vi "simulado.vi"() -> ()   [LabVIEW 2011]
uses:
  <vilib>/Simulation/Scripting/Companion Diagram/SimConfigNode/SimParams.ctl
  <vilib>/Simulation/Scripting/Companion Diagram/SimConfigNode/_simSolvers.ctl
  <vilib>/Simulation/Implementation/Shared/SIMSCR Execution Mode.ctl
  <vilib>/Simulation/Param Hierarchy/Typedefs/SIMPH Param Control Actions.ctl
  <vilib>/Simulation/Implementation/Shared/NILVSim_FinalizeModel.vi
  <vilib>/Simulation/DiscreteLinear/Implementation/NILVSim Discrete Transfer Function Direct.llb/SIM Discrete Transfer Function Direct (SISO CD).vi
  <vilib>/Simulation/DiscreteLinear/Implementation/NILVSim Discrete ZOH.llb/SIM Discrete ZOH (scalar).vi
  <vilib>/Simulation/Nonlinear/Implementation/NILVSim Saturation.llb/SIM Saturation (scalar).vi
  <vilib>/Simulation/SignalDisplay/Implementation/NILVSim Time Waveform.llb/SIM Time Waveform (vector).vi
  <vilib>/Simulation/Utility/Implementation/SIM Halt.vi
  <vilib>/Simulation/ContinuousLinear/Implementation/NILVSim Transfer Function.llb/SIM Transfer Function Collector (SISO).vi
  <vilib>/Simulation/ContinuousLinear/Implementation/NILVSim Transfer Function.llb/SIM Transfer Function Distributor (SISO CD).vi
  <vilib>/Simulation/Implementation/Shared/NILVSim_Manager.vi
  <vilib>/Simulation/Implementation/Shared/NILVSim_ParamChanged.vi
  <vilib>/Simulation/Utility/Implementation/NILVSim Get Time and IsAcceptedStep.vi
  <vilib>/addons/Control Design/_Model Construction/Model Creation.llb/Model Creation SubVI/cd_Create Transfer Function Model.vi
  <vilib>/addons/Control Design/_Utility/Model Viewer.llb/Model Viewer SubVI/cd_Draw Transfer Function Equation (TF).vi
  <vilib>/Simulation/Implementation/Shared/SIM Unbundle Sim Info.vi
  <vilib>/Simulation/Implementation/Shared/NILVSim_GetModelError.vi
  <vilib>/Simulation/Implementation/Shared/SIM Bundle Sim Info.vi
  <vilib>/Simulation/Implementation/Shared/NILVSim_Initialize.vi
  <vilib>/Simulation/Scripting/Companion Diagram/SimConfigNode/SimDog.xnode
  <vilib>/Simulation/Implementation/XNodeFramework/SimXNode/SimX.xnode
  <vilib>/addons/Control Design/_Model Construction/Model Typedefs.llb/CD Transfer Function Model (MIMO).ctl
  <vilib>/addons/Control Design/_Model Construction/Model Typedefs.llb/CD General Elements.ctl
  <vilib>/addons/Control Design/_Model Construction/Model Typedefs.llb/CD Transfer Function Model (SISO).ctl
  <vilib>/addons/Control Design/_Model Construction/NI_LinSys_Model Creation.lvlib
  <vilib>/addons/Control Design/_Utility/NI_CD_Model Viewer.lvlib
  <vilib>/addons/Control Design/_Model Construction/NI_LinSys_Model Typedefs.lvlib
  <vilib>/Simulation/ContinuousLinear/Implementation/NILVSim Transfer Function.llb/SIM Transfer Function (SISO CD).vi
  <vilib>/Simulation/Implementation/Shared/NI_SIM_Implementation.lvlib
panel:
  out "D(z)":picture
  out "P(s)":picture
  in  "Boolean":bool
  in  "Delay":dbl(knob)=0.01 scale=0.0..1.0
  out "?":waveform(dbl)[](graph)=[{"t0"=timestamp(8.4 s since 1904-01-01), "dt"=1.0, "Y"=[4.846938775510176]}, {"t0"=timestamp(8.4 s since 1904-01-01), "dt"=1.0, "Y"=[4.846938775510204]}]
  in  "Periodo muestreo (s)":dbl=0.03
  in  "Set Point":dbl(slide)=4.846938775510204 scale=0.0..5.0
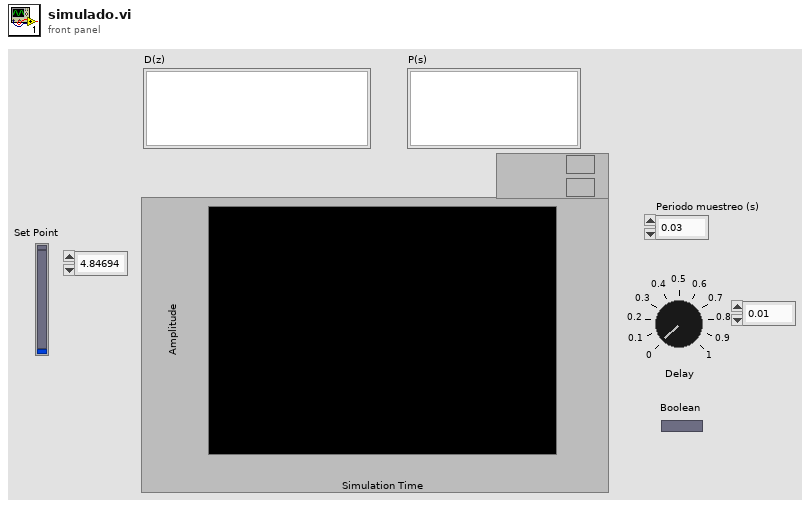
[diagram p1: front panel]
types:
  T1 = typedef "NI_LinSys_Model Typedefs.lvlib/CD Transfer Function Model (MIMO).ctl" = cluster{"properties":T2, "transfer function(s)":T3[][]}
  T2 = typedef "NI_LinSys_Model Typedefs.lvlib/CD General Elements.ctl" = cluster{"Model name":string, "Input names":string[], "Output names":string[], "Input Delays":dbl[], "Output Delays":dbl[], "Sampling Time":dbl, "Notes":string}
  T3 = typedef "NI_LinSys_Model Typedefs.lvlib/CD Transfer Function Model (SISO).ctl" = cluster{"Numerator":dbl[], "Denominator":dbl[], "delay":dbl}
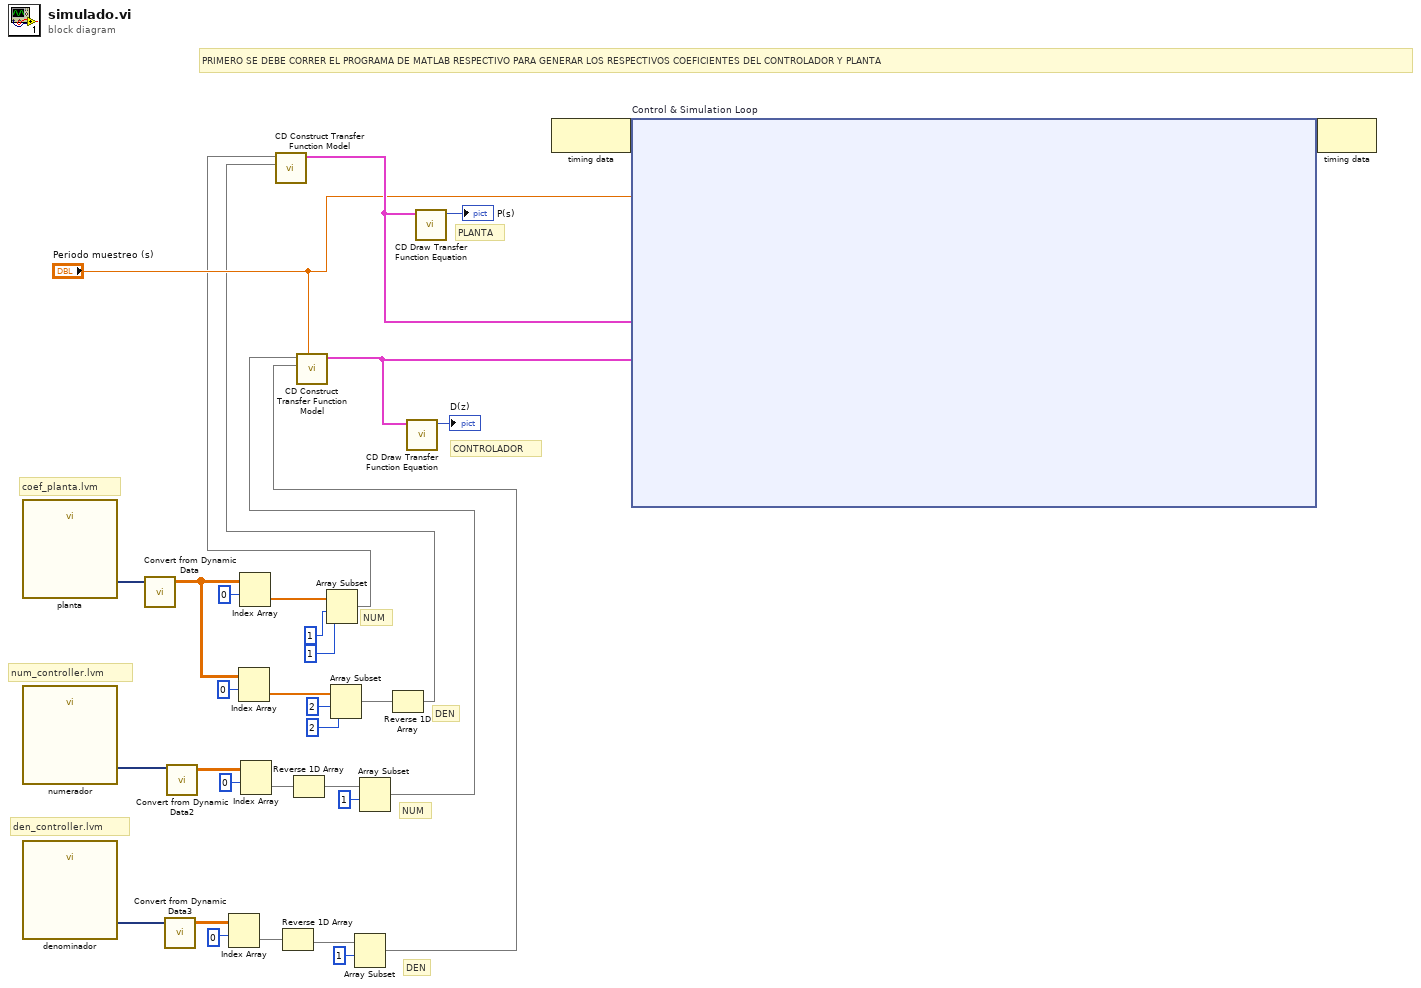
[diagram p0: block diagram]
diagram:
  # "DEN"
  # "NUM"
  # "DEN"
  # "NUM"
  # "PRIMERO SE DEBE CORRER EL PROGRAMA DE MATLAB RESPECTIVO PARA GENERAR LOS RESPECTIVOS COEFICIENTES DEL CONTROLADOR Y PLANTA"
  # "CONTROLADOR"
  # "den_controller.lvm"
  # "num_controller.lvm"
  # "coef_planta.lvm"
  # "PLANTA"
  n1 = call "planta"() -> ("Signals"=w27:dynamicdata)  [unwired: 6 in, 5 out]
  n2 = call "numerador"() -> ("Signals"=w4:dynamicdata)  [unwired: 6 in, 5 out]
  n3 = call "denominador"() -> ("Signals"=w2:dynamicdata)  [unwired: 6 in, 5 out]
  n4 = call "Convert from Dynamic Data"("Dynamic Data Type"=w27) -> ("Array"=w17:dbl[][])  [unwired: 3 in]
  n5 = call "Convert from Dynamic Data3"("Dynamic Data Type"=w2) -> ("Array"=w8:dbl[][])  [unwired: 3 in]
  n6 = call "Convert from Dynamic Data2"("Dynamic Data Type"=w4) -> ("Array"=w15:dbl[][])  [unwired: 3 in]
  n7 = Index Array(array=w8, index (row)=0) -> (element=w9:dbl[])  [unwired: 1 in]
  n8 = Index Array(array=w17, index (row)=0) -> (element=w19:dbl[])  [unwired: 1 in]
  n9 = Index Array(array=w17, index (row)=0) -> (element=w25:dbl[])  [unwired: 1 in]
  n10 = Index Array(array=w15, index (row)=0) -> (element=w14:dbl[])  [unwired: 1 in]
  n11 = Reverse 1D Array(array=w9) -> (reversed array=w10:dbl[])
  n12 = Reverse 1D Array(array=w14) -> (reversed array=w13:dbl[])
  n13 = Array Subset(array=w25, index=1, length=1) -> (w6:dbl[])
  n14 = Array Subset(array=w19, index=2, length=2) -> (w18:dbl[])
  n15 = Array Subset(array=w10, index=1) -> (w1:dbl[])  [unwired: 1 in]
  n16 = Array Subset(array=w13, index=1) -> (w3:dbl[])  [unwired: 1 in]
  n17 = call-poly <vilib>:"CD Construct Transfer Function Model.vi"("Sampling Time (s)"="Periodo muestreo (s)", "Denominator"=w1, "Numerator"=w3) -> ("Transfer Function Model"=w32:T1)  [unwired: 7 in, 1 out]
  n18 = Reverse 1D Array(array=w18) -> (reversed array=w5:dbl[])
  n19 = call-poly <vilib>:"CD Construct Transfer Function Model.vi"("Denominator"=w5, "Numerator"=w6) -> ("Transfer Function Model"=w31:T1)  [unwired: 8 in, 1 out]
  n20 = call-poly <vilib>:"CD Draw Transfer Function Equation.vi"("Transfer Function Model"=w32) -> ("Equation"=→"D(z)":picture)  [unwired: 8 in, 2 out]
  n21 = call-poly <vilib>:"CD Draw Transfer Function Equation.vi"("Transfer Function Model"=w31) -> ("Equation"=→"P(s)":picture)  [unwired: 8 in, 2 out]
  n22 = node-c288() -> (w34:variant)  [unwired: 1 in]
  n23 = node-c254 "Control & Simulation Loop"(w34, w32, "Periodo muestreo (s)", w31) -> (w33:variant)
  n24 = node-c288(w33) -> ()  [unwired: 1 out]
